vi "Memory.Pointer.Read In Place.vi"(7 "length (-1: all)":i64=-1 format="%d bytes", 8 "error in (no error)":errorcluster, 9 "offset (0)":u64 format="%d bytes", 10 "data in":string, 11 "Pointer in":refnum<class "Memory.Pointer.lvclass">) -> (0 "error out":errorcluster, 1 "offset dup":u64 format="%d bytes", 2 "data out":string, 3 "Pointer out":refnum<class "Memory.Pointer.lvclass">)   [LabVIEW 2016, in "LabVIEW Memory Manager.lvlib" / "Memory.Pointer.lvclass"]
uses:
  Memory.Pointer.lvclass
  Memory.Pointer.lvclass/Memory.Pointer.ctl
  Accessors/Memory.Pointer.Get Address.vi
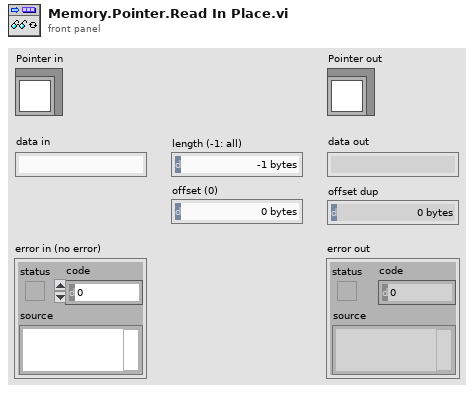
[diagram p1: front panel]
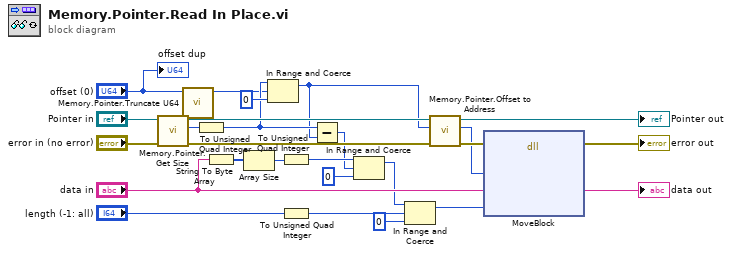
[diagram p0: block diagram]
diagram:
  n1 = call "Memory.Pointer.Get Size.vi"("error in (no error)"="error in (no error)", "Pointer in"="Pointer in") -> ("error out"=w25:errorcluster, "size"=w19:i64, "Pointer out"=w26:refnum<class "Memory.Pointer.lvclass">)  [unwired: 7 in]
  n2 = call "Memory.Pointer.Truncate U64.vi"("U64"="offset (0)") -> ("truncated U64"=w2:u64)  [unwired: 10 in]
  n3 = To Unsigned Quad Integer(1:w19) -> (0:w18:u64)
  n4 = String To Byte Array(string="data in") -> (unsigned byte array=w9:u8[])
  n5 = Array Size(array=w9) -> (size(s)=w6:i32)
  n6 = In Range and Coerce(upper limit=w18, x=w2, lower limit=u64 0) -> (coerced(x)=w17:u64)  [unwired: 1 out]
  n7 = To Unsigned Quad Integer(1:w6) -> (0:w5:u64)
  n8 = To Unsigned Quad Integer(1:"length (-1: all)") -> (0:w16:u64)
  n9 = Subtract(x=w18, y=w17) -> (x-y=w4:u64)
  n10 = In Range and Coerce(upper limit=w5, x=w4, lower limit=u64 0) -> (coerced(x)=w3:u64)  [unwired: 1 out]
  n11 = In Range and Coerce(upper limit=w3, x=w16, lower limit=u64 0) -> (coerced(x)=w24:u64)  [unwired: 1 out]
  n12 = call "Memory.Pointer.Offset to Address.vi"("error in (no error)"=w25, "offset"=w17, "Pointer in"=w26) -> ("error out"=w22:errorcluster, "offset address"=w21:u64, "Pointer out"=→"Pointer out":refnum<class "Memory.Pointer.lvclass">)  [unwired: 6 in]
  n13 = dll-call lib="LabVIEW" fn="MoveBlock"(error in=w22, "src pointer"=w21, "dst pointer"="data in", "size"=w24) -> (error out=→"error out":errorcluster, "dst pointer"=→"data out":string)  [unwired: 5 in, 1 out]
  "offset dup" <- "offset (0)"
